vi "Init Actor Core.vi"(8 "error in (no error)":errorcluster, 11 "Measure Object in":refnum<class "Application Controller.lvclass">) -> (0 "error out":errorcluster, 3 "Measure Object out":refnum<class "Application Controller.lvclass">)   [LabVIEW 2018, in "Application Controller.lvclass"]
uses:
  Application Controller.lvclass
  C:/github/2018/LabActor/Template Module/Template Module.lvclass
  C:/Program Files/National Instruments/LabVIEW 2018/vi.lib/ActorFramework/Actor/Actor.lvclass
  Application Controller.lvclass/Application Controller.ctl
  Template Module/Template Module.lvclass/Template Module.ctl
  <vilib>/ActorFramework/Actor/Actor.lvclass/Actor.ctl
  <vilib>/ActorFramework/Message Enqueuer/Message Enqueuer.lvclass/Message Enqueuer.ctl
  Read Launch Notifier.vi
  Template Module/Read Name.vi
  Read Start-up configuration file.vi
  <vilib>/ActorFramework/Message Enqueuer/Enqueue.vi
  <vilib>/ActorFramework/Message Enqueuer/Init from Existing Queue.vi
  Comms/Communications Messages/Init Comms Msg/Init Comms Msg.lvclass
  C:/Program Files/National Instruments/LabVIEW 2018/vi.lib/ActorFramework/Message/Message.lvclass
  Application Controller Messages/Load Complete Msg/Load Complete Msg.lvclass
  <vilib>/ActorFramework/Message Priority Queue/Priority Enqueue.vi
  <vilib>/ActorFramework/Message Enqueuer/Message Enqueuer.lvclass
  Process Controller/Process Controller.lvclass
  <vilib>/ActorFramework/Actor/Actor.lvclass
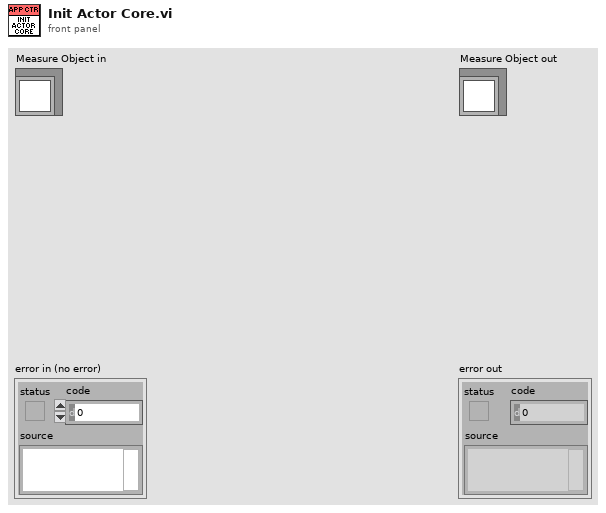
[diagram p1: front panel]
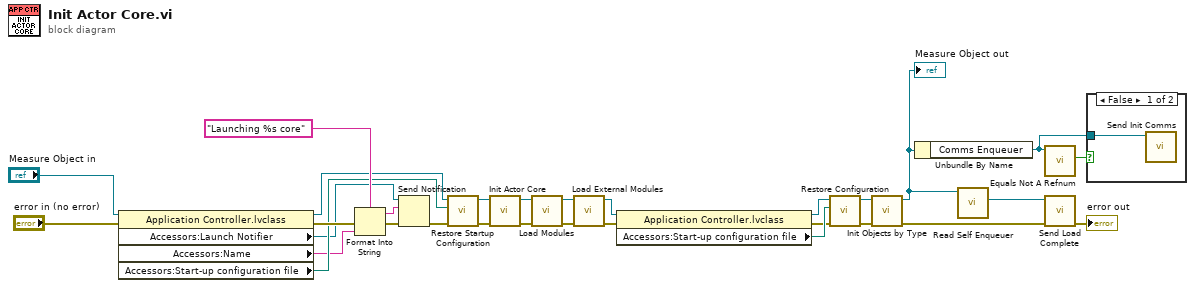
[diagram p0: block diagram]
diagram:
  n1 = property class="Application Controller.lvclass"(reference="Measure Object in", error in="error in (no error)") -> (reference out=w25:refnum<class "Application Controller.lvclass">, error out=w27:errorcluster, "Accessors:Launch Notifier"=w16:refnum<notifier>, "Accessors:Name"=w17:string, "Accessors:Start-up configuration file"=w18:path)
  n2 = Format Into String(format string="Launching %s core" ("notification"), error in=w27, w17) -> (resulting string=w15:string, error out=w26:errorcluster)  [unwired: 1 in]
  n3 = Send Notification(notification=w15, notifier=w16, error in (no error)=w26) -> (error out=w24:errorcluster)  [unwired: 1 out]
  n4 = call-dynamic "Restore Startup Configuration.vi"("error in (no error)"=w24, "Startup Configuration File"=w18, "Monitor-Pulse in"=w25) -> ("error out"=w22:errorcluster, "Monitor-Pulse out"=w19:refnum<class "Application Controller.lvclass">)  [unwired: 6 in, 1 out]
  n5 = call-parent "Init Actor Core.vi"("error in (no error)"=w22, "Measure Object in"=w19) -> ("error out"=w21:errorcluster, "Measure Object out"=w13:refnum<class "Application Controller.lvclass">)  [unwired: 8 in]
  n6 = call-dynamic "Load Modules.vi"("error in (no error)"=w21, "Application Controller in"=w13) -> ("error out"=w4:errorcluster, "Application Controller out"=w3:refnum<class "Application Controller.lvclass">)  [unwired: 8 in]
  n7 = call-dynamic "Load External Modules.vi"("error in (no error)"=w4, "Application Controller in"=w3) -> ("error out"=w2:errorcluster, "Application Controller out"=w1:refnum<class "Application Controller.lvclass">)  [unwired: 8 in]
  n8 = property class="Application Controller.lvclass"(reference=w1, error in=w2) -> (reference out=w12:refnum<class "Application Controller.lvclass">, error out=w10:errorcluster, "Accessors:Start-up configuration file"=w11:path)
  n9 = call-dynamic "Restore Configuration.vi"("error in (no error)"=w10, "File path"=w11, "Measure Object in"=w12) -> ("error out"=w9:errorcluster, "Measure Object out"=w8:refnum<class "Application Controller.lvclass">)  [unwired: 5 in, 2 out]
  n10 = call-dynamic "Init Objects by Type.vi"("error in (no error)"=w9, "Application Controller in"=w8) -> ("error out"=w14:errorcluster, "Application Controller out"=w7:refnum<class "Application Controller.lvclass">)  [unwired: 8 in]
  "Measure Object out" <- w7
  n11 = Unbundle By Name(w7) -> ("Comms Enqueuer"=w6:refnum<class "Message Enqueuer.lvclass">)
  n12 = call <vilib>:"Read Self Enqueuer.vi"("Actor"=w7) -> ("Self Enqueuer"=w23:refnum<class "Message Enqueuer.lvclass">)  [unwired: 10 in]
  n13 = call <vilib>:"Equals Not A Refnum.vi"("Message Enqueuer"=w6) -> ("Not a refnum?"=w5:bool)  [unwired: 10 in]
  n14 = call "Send Load Complete.vi"("error in (no error)"=w14, "Message Enqueuer"=w23) -> ("error out"=→"error out":errorcluster)  [unwired: 8 in, 1 out]
  n15 = case shown="False" w5 {
    tunnel: w6 -> [w31 _]
    frame False {
      n16 = call "Send Init Comms.vi"("Message Enqueuer"=w31) -> ()  [unwired: 9 in, 2 out]
    }
    frame True {
    }
  }
